vi "BuildHologram.vi"(9 "Hologram array":dbl[](array[numeric])=[0.0, 0.25, 0.5, 0.75], 11 "Array":dbl[](array[numeric])) -> (3 "hologram":cdb)   [LabVIEW 2018, in "Photon Filtering.lvlib"]
uses:
  Photon Filtering.lvlib
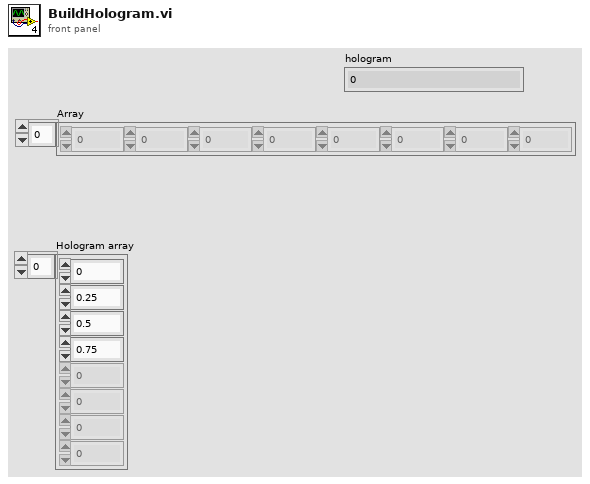
[diagram p1: front panel]
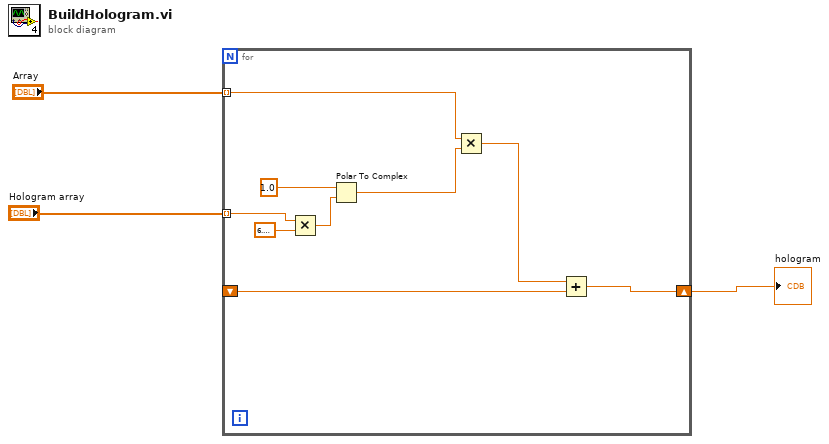
[diagram p0: block diagram]
diagram:
  n1 = for {
    tunnel: "Array" -> [w8] mode=indexing
    tunnel: "Hologram array" -> [w11] mode=indexing
    shift-right: [w5] -> w1
    shift-left: _ -> [w4]
    n2 = Multiply(x=w11, y=6.283185307179586) -> (x*y=w9:dbl)
    n3 = Polar To Complex(1:w9, 2:1.0 ("r")) -> (0:w7:cdb)
    n4 = Multiply(x=w8, y=w7) -> (x*y=w6:cdb)
    n5 = Add(x=w6, y=w4) -> (x+y=w5:cdb)
  }
  "hologram" <- w1
